vi "Delay Fix.vi"() -> ()   [LabVIEW 2024]
panel:
  out "Cycles":dbl format="%#_6p"
  in  "Stop Button":bool
  in  "Delay":dbl step=1e-09 format="%#_6ps"
  out "XY Graph":cluster{dbl[], dbl[]}[](graph)
  in  "Channels":string[](array[string])=["Frequency", "Signal X", "Signal Y"]
  in  "Group":string="p"
  in  "File Path Control":path=path "C:/Data/October_2018/101618/sp0003_101618.tdms"
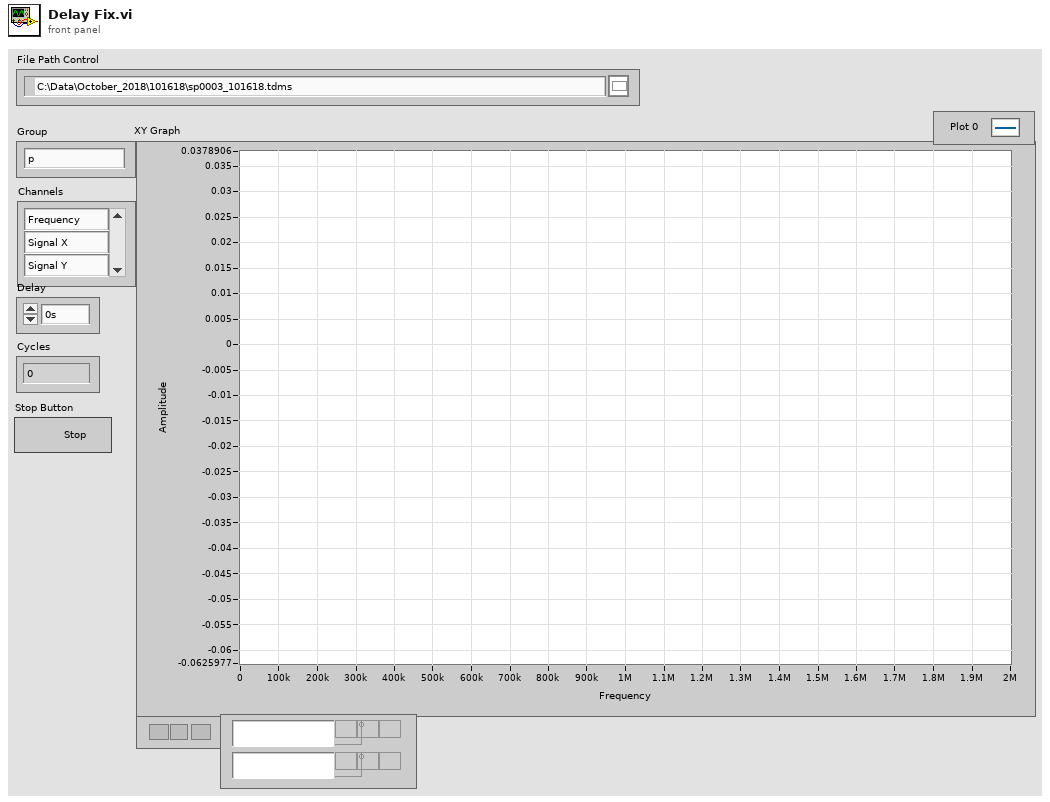
[diagram p1: front panel]
types:
  T1 = enum16{"open", "open or create", "create or replace", "create", "open (read-only)"}
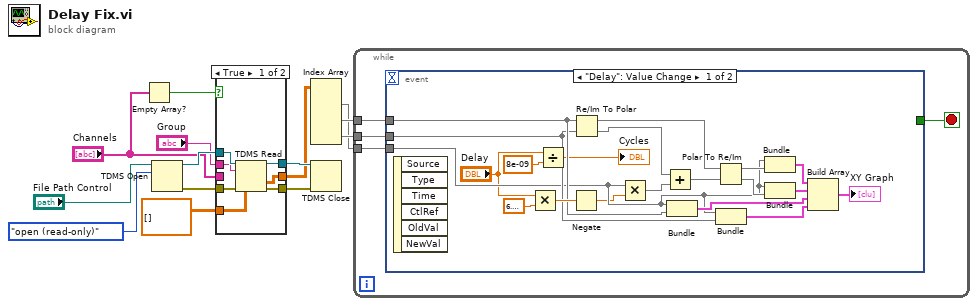
[diagram p0: block diagram]
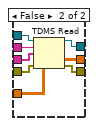
[diagram p2: hidden frame]
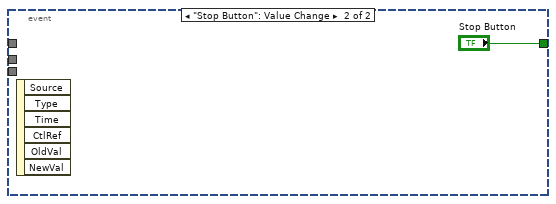
[diagram p3: hidden frame]
diagram:
  n1 = Empty Array?(array="Channels") -> (empty?=w1:bool)
  n2 = TDMS Open(10:T1."open (read-only)" ("operation (0:open)"), 11:"File Path Control") -> (0:w11:errorcluster, 3:w12:refnum<k34>)  [unwired: 5 in]
  n3 = case shown="True" w1 {
    tunnel: w12 -> [w21 w29]
    tunnel: w11 -> [w20 w28]
    tunnel: "Group" -> [w19 w27]
    tunnel: "Channels" -> [_ w26]
    tunnel: [w18 w25] -> w9
    tunnel: [w17 w24] -> w8
    tunnel: dbl[][] [] -> [w16 w23]
    tunnel: [w15 w22] -> w6
    frame True {
      n4 = TDMS Read(0:w21, 5:w19, 11:w20, 12:w16) -> (4:w17:refnum<k34>, 10:w15:dbl[][], 15:w18:errorcluster)  [unwired: 4 in, 3 out]
    }
    frame False {
      n5 = TDMS Read(0:w29, 5:w27, 7:w26, 11:w28, 12:w23) -> (4:w24:refnum<k34>, 10:w22:dbl[][], 15:w25:errorcluster)  [unwired: 3 in, 3 out]
    }
  }
  n6 = Index Array(array=w6) -> (element #1=w3:dbl[], element #2=w5:dbl[], element #3=w4:dbl[])  [unwired: 6 in]
  n7 = TDMS Close(8:w9, 11:w8) -> ()  [unwired: 2 out]
  n8 = while {
    tunnel: w5 -> [w33]
    tunnel: w4 -> [w32]
    tunnel: w3 -> [w31]
    stop <- w30 stop-if-true
    n9 = event shown="[0] \"Delay\": Value Change" {
      selector: _ -> [_ _]
      dyn-events: _ -> [_ _]
      timeout: _ -> [_ _]
      tunnel: w33 -> [w48 _]
      tunnel: w32 -> [w47 _]
      tunnel: w31 -> [w40 _]
      tunnel: [_ "Stop Button"] -> w30
      event "Delay": Value Change {
        n10 = event-data() -> ()  [unwired: 1 in, 6 out]
        n11 = Multiply(x="Delay", y=6.283185307179586) -> (x*y=w49:dbl)
        n12 = Divide(x="Delay", y=8e-09) -> (x/y=→"Cycles":dbl)
        n13 = Negate(x=w49) -> (-x=w34:dbl)
        n14 = Re/Im To Polar(2:w47, 3:w48) -> (0:w46:dbl[], 1:w43:dbl[])
        n15 = Multiply(x=w40, y=w34) -> (x*y=w45:dbl[])
        n16 = Add(x=w46, y=w45) -> (x+y=w44:dbl[])
        n17 = Bundle(w40, w48) -> (w53:cluster{dbl[], dbl[]})  [unwired: 1 in]
        n18 = Polar To Re/Im(2:w44, 3:w43) -> (0:w41:dbl[], 1:w42:dbl[])
        n19 = Bundle(w40, w47) -> (w52:cluster{dbl[], dbl[]})  [unwired: 1 in]
        n20 = Bundle(w40, w42) -> (w39:cluster{dbl[], dbl[]})  [unwired: 1 in]
        n21 = Bundle(w40, w41) -> (w38:cluster{dbl[], dbl[]})  [unwired: 1 in]
        n22 = Build Array(w39, w38, w53, w52) -> (→"XY Graph":cluster{dbl[], dbl[]}[])
      }
      event "Stop Button": Value Change {
        n23 = event-data() -> ()  [unwired: 1 in, 6 out]
      }
    }
  }
